vi "Read Worker.vi"(8 "error in (no error)":errorcluster, 11 "Chef State in":refnum<class "Chef State.lvclass">) -> (0 "error out":errorcluster, 3 "Chef State out":refnum<class "Chef State.lvclass">)   [LabVIEW 2024]
uses:
  Chef State.lvclass
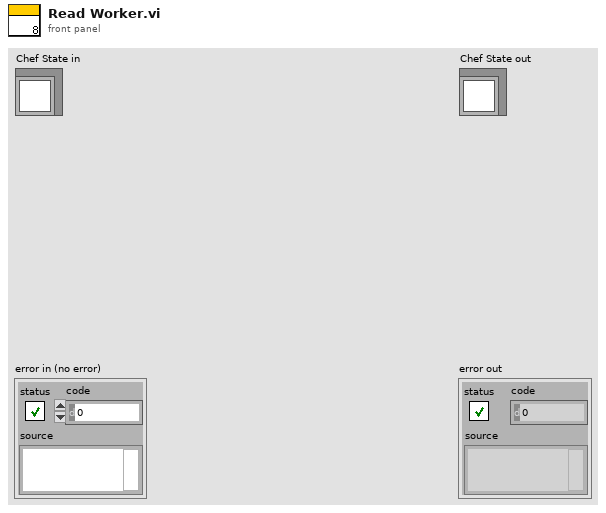
[diagram p1: front panel]
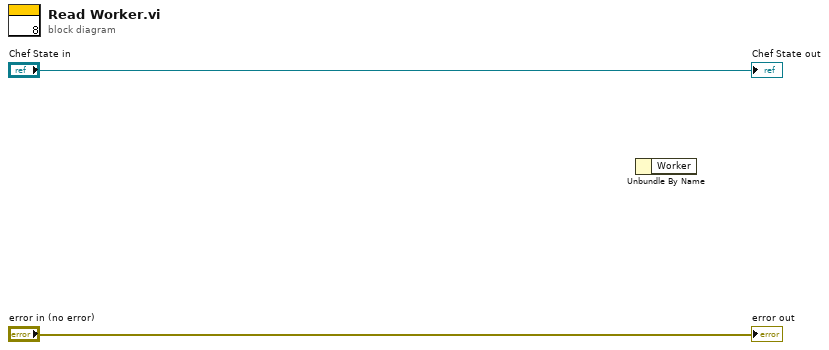
[diagram p0: block diagram]
diagram:
  n1 = Unbundle By Name() -> ()  [unwired: 1 in, 1 out]
  "error out" <- "error in (no error)"
  "Chef State out" <- "Chef State in"
